vi "Counts Update.vi"(5 "Perf":T1, 6 "output cluster":T3, 7 "Cluster":cluster{"Time":timestamp, "Auto Times":T2}, 8 "Desired Cycle Time (s)":dbl=2.0, 9 "AVL":dbl=100.0 min=0.0 max=100.0 step=0.1, 10 "OutputCount":u32, 11 "Counts in":cluster{"OutputCount":u32, "RejectCount":u32}) -> (1 "OEE":T5={"AVL"=100.0, "PRF"=100.0, "QUA"=100.0, "OEE"=0.0} {"OEE" format="%#.1f"; "QUA" min=0.0 max=100.0 step=0.1; "PRF" min=0.0 max=100.0 step=0.1; "AVL" min=0.0 max=100.0 step=0.1}, 2 "Auto Stats":T4={"Time"=timestamp(0 s since 1904-01-01), "OEE"={"AVL"=100.0, "PRF"=100.0, "QUA"=100.0, "OEE"=0.0}, "Auto Times"={"Index Time"=0, "TF Time"=0, "Insertion Time"=0, "Cutting Time"=0, "PF Time"=0, "Meas. Time"=0, "Reject Time"=0}, "Counts out"={"OutputCount"=0, "RejectCount"=0}, "Measurements"={"1"=0.0, "2"=0.0, "3"=0.0, "4"=0.0}, "Outputs"={"OutputCount"=0, "Numeric Control"=0}} {"OEE"."OEE" format="%#.1f"; "OEE"."QUA" min=0.0 max=100.0 step=0.1; "OEE"."PRF" min=0.0 max=100.0 step=0.1; "OEE"."AVL" min=0.0 max=100.0 step=0.1}, 3 "Counts out":cluster{"OutputCount":u32, "RejectCount":u32})   [LabVIEW 2017]
uses:
  support/Controls/Auto Stats.ctl
  RT/Controls/Auto Times.ctl
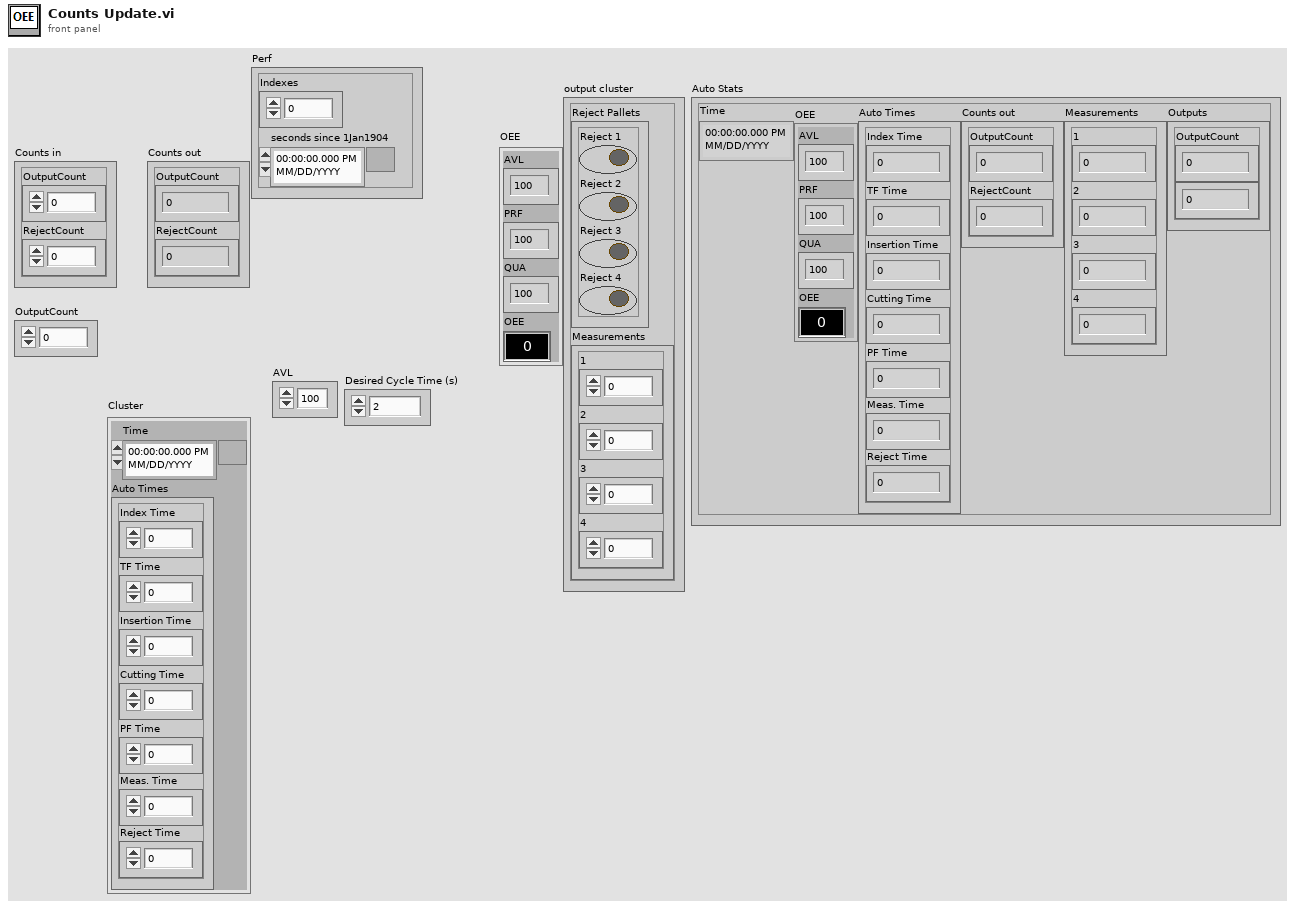
[diagram p1: front panel]
types:
  T1 = cluster{"Indexes":i32, "seconds since 1Jan1904":timestamp}
  T2 = typedef "Auto Times.ctl" = cluster{"Index Time":u32, "TF Time":u32, "Insertion Time":u32, "Cutting Time":u32, "PF Time":u32, "Meas. Time":u32, "Reject Time":u32}
  T3 = cluster{"Reject Pallets":cluster{"Reject 1":bool, "Reject 2":bool, "Reject 3":bool, "Reject 4":bool}, "Measurements":cluster{"1":dbl, "2":dbl, "3":dbl, "4":dbl}}
  T4 = typedef "Auto Stats.ctl" = cluster{"Time":timestamp, "OEE":cluster{"AVL":dbl, "PRF":dbl, "QUA":dbl, "OEE":dbl}, "Auto Times":T2, "Counts out":cluster{"OutputCount":u32, "RejectCount":u32}, "Measurements":cluster{"1":dbl, "2":dbl, "3":dbl, "4":dbl}, "Outputs":cluster{"OutputCount":u32, "Numeric Control":u32}}
  T5 = cluster{"AVL":dbl, "PRF":dbl, "QUA":dbl, "OEE":dbl}
  T6 = cluster{"Reject 1":bool, "Reject 2":bool, "Reject 3":bool, "Reject 4":bool}
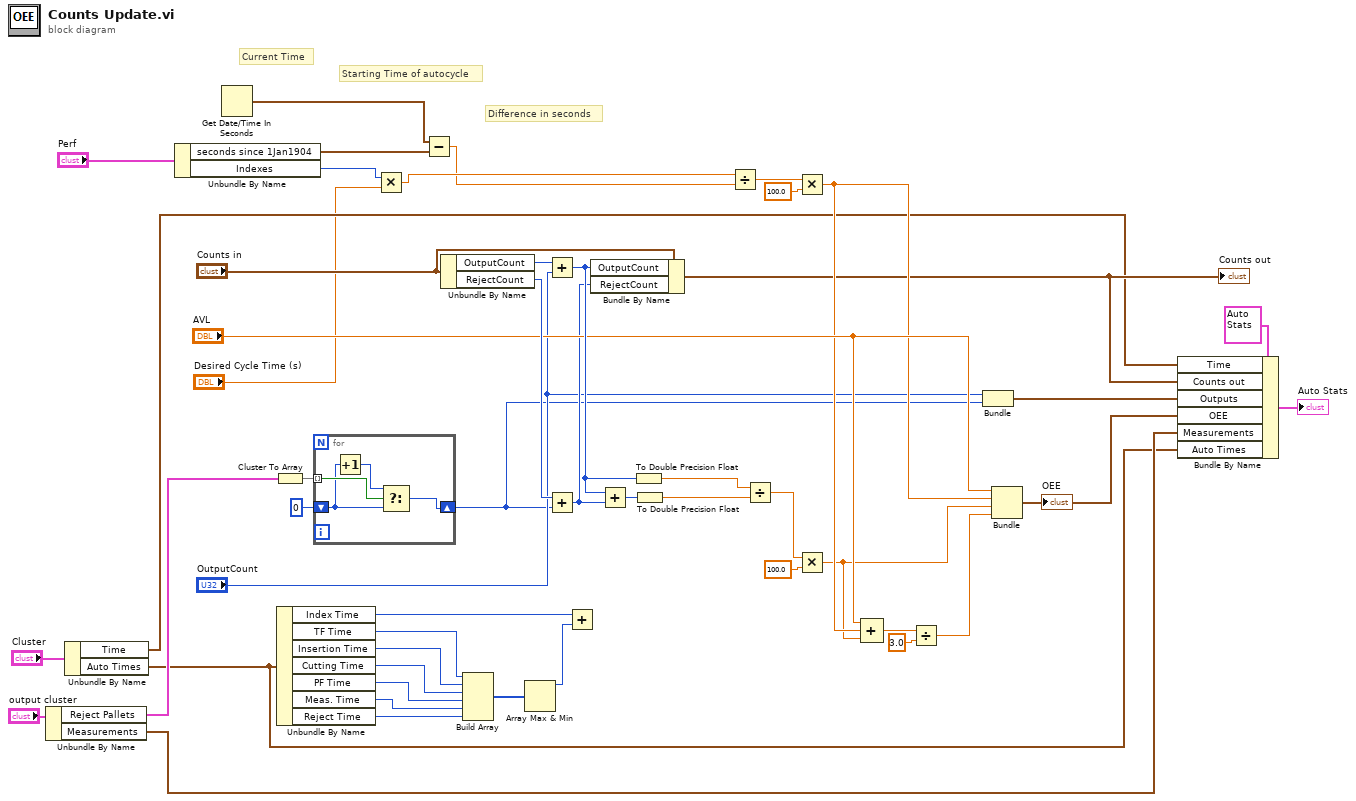
[diagram p0: block diagram]
diagram:
  # "Difference in seconds"
  # "Starting Time of autocycle"
  # "Current Time"
  n1 = Unbundle By Name("output cluster") -> ("Reject Pallets"=w11:T6, "Measurements"=w12:cluster{"1":dbl, "2":dbl, "3":dbl, "4":dbl})
  n2 = Unbundle By Name("Cluster") -> ("Time"=w8:timestamp, "Auto Times"=w9:T2)
  n3 = Unbundle By Name("Perf") -> ("seconds since 1Jan1904"=w5:timestamp, "Indexes"=w3:i32)
  n4 = Get Date/Time In Seconds() -> (seconds since 1Jan1904=w6:timestamp)
  n5 = Cluster To Array(cluster=w11) -> (array=w47:bool[])
  n6 = Unbundle By Name(w9) -> ("Index Time"=w38:u32, "TF Time"=w32:u32, "Insertion Time"=w33:u32, "Cutting Time"=w34:u32, "PF Time"=w35:u32, "Meas. Time"=w36:u32, "Reject Time"=w37:u32)
  n7 = for {
    tunnel: w47 -> [w53] mode=indexing
    shift-right: [w52] -> w19
    shift-left: u32 0 -> [w51]
    n8 = Increment(x=w51) -> (x+1=w50:u32)
    n9 = Select(t=w50, s=w53, f=w51) -> (s? t:f=w52:u32)
  }
  n10 = Multiply(x=w3, y="Desired Cycle Time (s)") -> (x*y=w2:dbl)
  n11 = Subtract(x=w6, y=w5) -> (x-y=w1:dbl)
  n12 = Unbundle By Name("Counts in") -> ("OutputCount"=w49:u32, "RejectCount"=w48:u32)
  n13 = Build Array(w32, w33, w34, w35, w36, w37) -> (w31:u32[])
  n14 = Array Max & Min(array=w31) -> (max value=w30:u32)  [unwired: 3 out]
  n15 = Add(x=w49, y="OutputCount") -> (x+y=w43:u32)
  n16 = Add(x=w48, y=w19) -> (x+y=w21:u32)
  n17 = Add(x=w38, y=w30) -> ()  [unwired: 1 out]
  n18 = Bundle By Name(cluster="Counts in", "OutputCount"=w43, "RejectCount"=w21) -> (w15:cluster{"OutputCount":u32, "RejectCount":u32})
  "Counts out" <- w15
  n19 = Add(x=w43, y=w21) -> (x+y=w44:u32)
  n20 = To Double Precision Float(number=w43) -> (double precision float=w23:dbl)
  n21 = To Double Precision Float(number=w44) -> (double precision float=w22:dbl)
  n22 = Divide(x=w2, y=w1) -> (x/y=w28:dbl)
  n23 = Divide(x=w23, y=w22) -> (x/y=w41:dbl)
  n24 = Multiply(x=w28, y=100.0) -> (x*y=w25:dbl)
  n25 = Multiply(x=w41, y=100.0) -> (x*y=w24:dbl)
  n26 = Compound Arithmetic op=ADD("AVL", w25, w24) -> (w42:dbl)
  n27 = Divide(x=w42, y=3.0) -> (x/y=w26:dbl)
  n28 = Bundle("OutputCount"="OutputCount", w19) -> (w17:cluster{"OutputCount":u32, u32})  [unwired: 1 in]
  n29 = Bundle("AVL"="AVL", w25, w24, w26) -> (w16:cluster{"AVL":dbl, dbl, dbl, dbl})  [unwired: 1 in]
  "OEE" <- w16
  n30 = Bundle By Name(cluster=T4 {"Time"=timestamp(0 s since 1904-01-01), "OEE"={"AVL"=100.0, "PRF"=100.0, "QUA"=100.0, "OEE"=0.0}, "Auto Times"={"Index Time"=0, "TF Time"=0, "Insertion Time"=0, "Cutting Time"=0, "PF Time"=0, "Meas. Time"=0, "Reject Time"=0}, "Counts out"={"OutputCount"=0, "RejectCount"=0}, "Measurements"={"1"=0.0, "2"=0.0, "3"=0.0, "4"=0.0}, "Outputs"={"OutputCount"=0, "Numeric Control"=0}} ("Auto Stats"), "Time"=w8, "Counts out"=w15, "Outputs"=w17, "OEE"=w16, "Measurements"=w12, "Auto Times"=w9) -> (→"Auto Stats":T4)
